vi "Funct TIFF export-Abort export.vi"   [LabVIEW 2020]
uses:
  Globals/gl_funct TIFF export globals.vi
types:
  T1 = typedef "Funct TIFF exporter ctrl refs.ctl" = cluster{"This VI":refnum<vi>, "Current Experiment":refnum<vi>, "Imaging protocol":refnum<vi>, "Predominant ROI type":refnum<vi>, "Patches in Experiment":refnum<vi>, "Folder Path":refnum<vi>, "Export":refnum<vi>, "Trial number":refnum<vi>, "Output TIFF type":refnum<vi>}
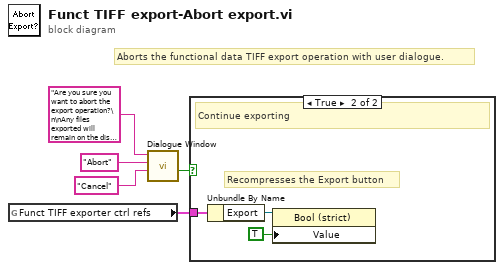
[diagram p0: block diagram]
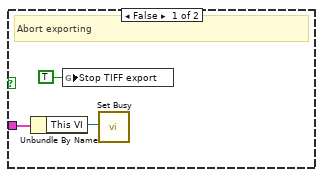
[diagram p2: hidden frame]
diagram:
  # "Aborts the functional data TIFF export operation with user dialogue."
  n1 = global read "gl_funct TIFF export globals.vi" "Funct TIFF exporter ctrl refs"() -> (w1:T1)
  n2 = call "Dialogue Window.vi"("Caption-Left button (Cancel)"="Cancel", "Caption-Right button (OK)"="Abort", "Message string"="Are you sure you want to abort the export operation?\n\nAny files exported will remain on the disk.\n") -> ("Cancelled (Left button pressed)"=w2:bool)  [unwired: 6 in, 2 out]
  n3 = case shown="True" w2 {
    tunnel: w1 -> [w6 w11]
    frame False {
      # "Abort exporting"
      n4 = Unbundle By Name(w6) -> ("This VI"=w8:refnum<vi>)
      n5 = global write "gl_funct TIFF export globals.vi" "Stop TIFF export"(TRUE ("Stop TIFF export")) -> ()
      n6 = call <vilib>:"Set Busy.vi"("VI reference (current VI)"=w8) -> ()  [unwired: 9 in, 2 out]
    }
    frame True {
      # "Recompresses the Export button"
      # "Continue exporting"
      n7 = Unbundle By Name(w11) -> ("Export"=w10:refnum<vi>)
      n8 = property class="Bool (strict)"(reference=w10, "Value"=TRUE) -> ()  [unwired: 1 in, 2 out]
    }
  }
